vi "Realtime Monitor.vi"() -> ()   [LabVIEW 2020]
uses:
  <vilib>/Utility/sysdir.llb/System Directory Type.ctl
  <vilib>/Utility/error.llb/DialogType.ctl
  global/GlobalVariable.vi
  global/SettingVariable.vi
  <vilib>/Analysis/polynomials.llb/Scalar Polynomial Evaluation (DBL).vi
  <vilib>/Analysis/NI_AALPro.lvlib
panel:
  out "T2周期":dbl[](array[numeric]) caption="倍增周期 (s):"
  in  "拟合数":i32(knob)=5 scale=5.0..100.0
  out "实时监测趋势图":dbl[][](graph) caption="Waveform Chart - Dark"
  in  "量程衔接 2":bool
  out "量程衔接开":bool
  out "四路VO":dbl[](array[numeric]) caption="四路电压输出(V)："
  out "反应性OUT":dbl[](array[numeric])
  out "源与本底开":bool
  in  "源与本底":bool
  out "滤波开":bool
  in  "通量滤波":bool
  out "DRWM开":bool
  in  "动态刻棒":bool
  in  "量程衔接":bool
  in  "添加备注说明":string caption="添加备注说明："
  in  "Start Button":bool
  in  "停止测量":bool
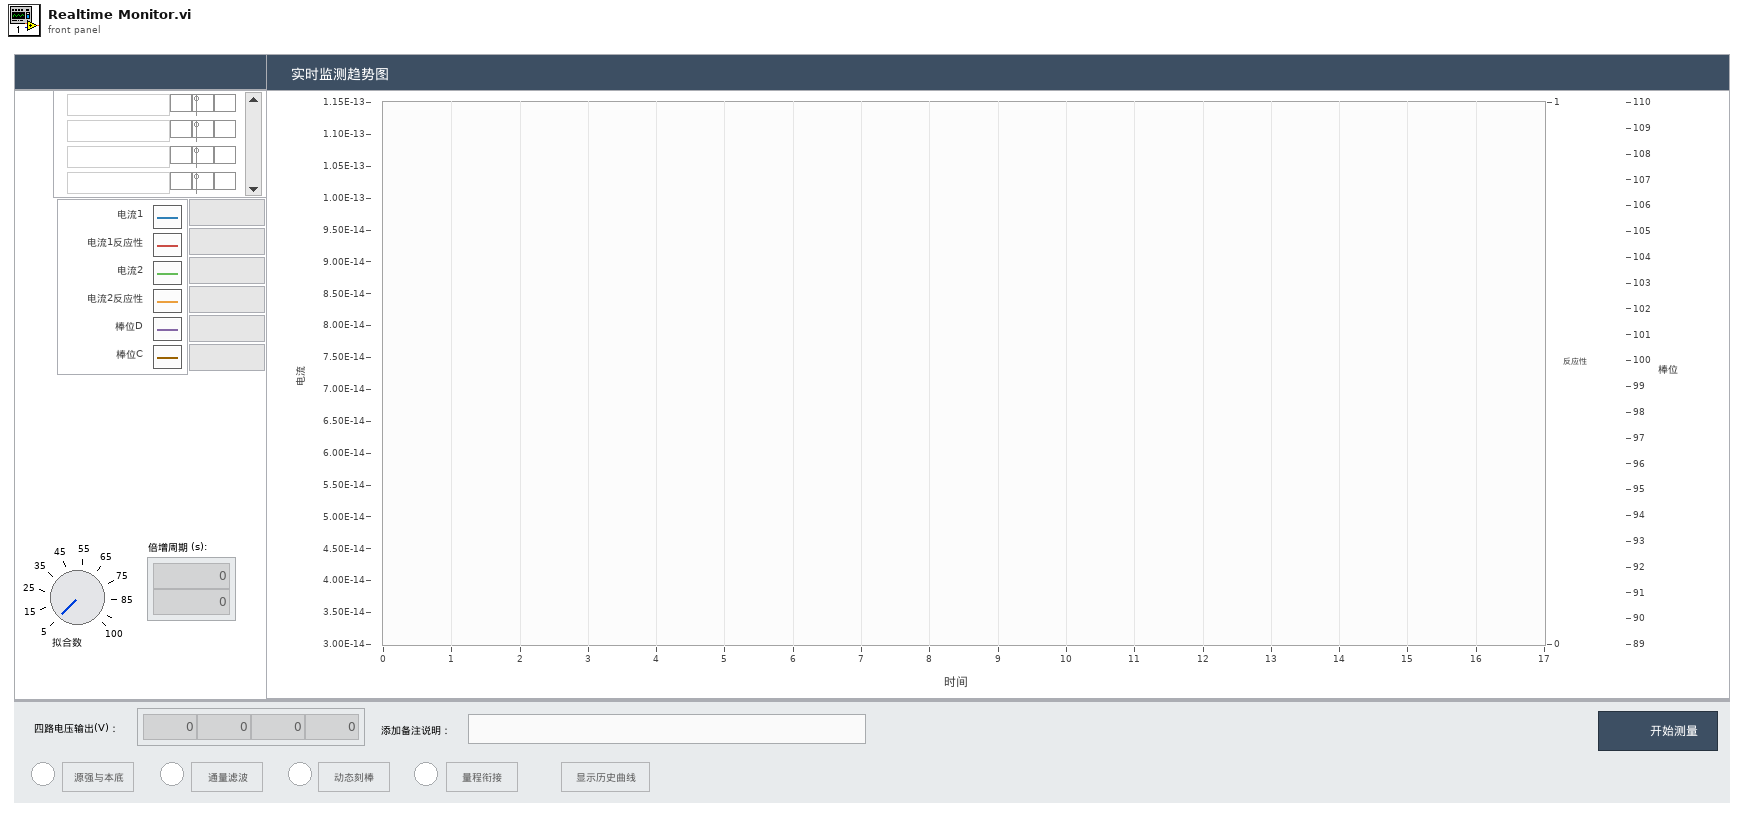
[diagram p1: front panel]
types:
  T1 = enum8{"Enabled", "Disabled", "Disabled and Grayed Out"}
  T2 = enum16{"open", "open or create", "create or replace", "create", "open (read only)"}
  T3 = cluster{"switch":bool, "name":string, "voltage upper":i32, "voltage lower":i32, "physics upper":dbl, "physics lower":dbl, "scale":u16}[]
  T4 = typedef "DialogType.ctl" = u16
  T5 = typedef "System Directory Type.ctl" = i32
  T6 = cluster{"switch":bool, "voltage upper":i32, "voltage lower":i32, "physics upper":dbl, "physics lower":dbl, "input":u16, "log":bool}[]
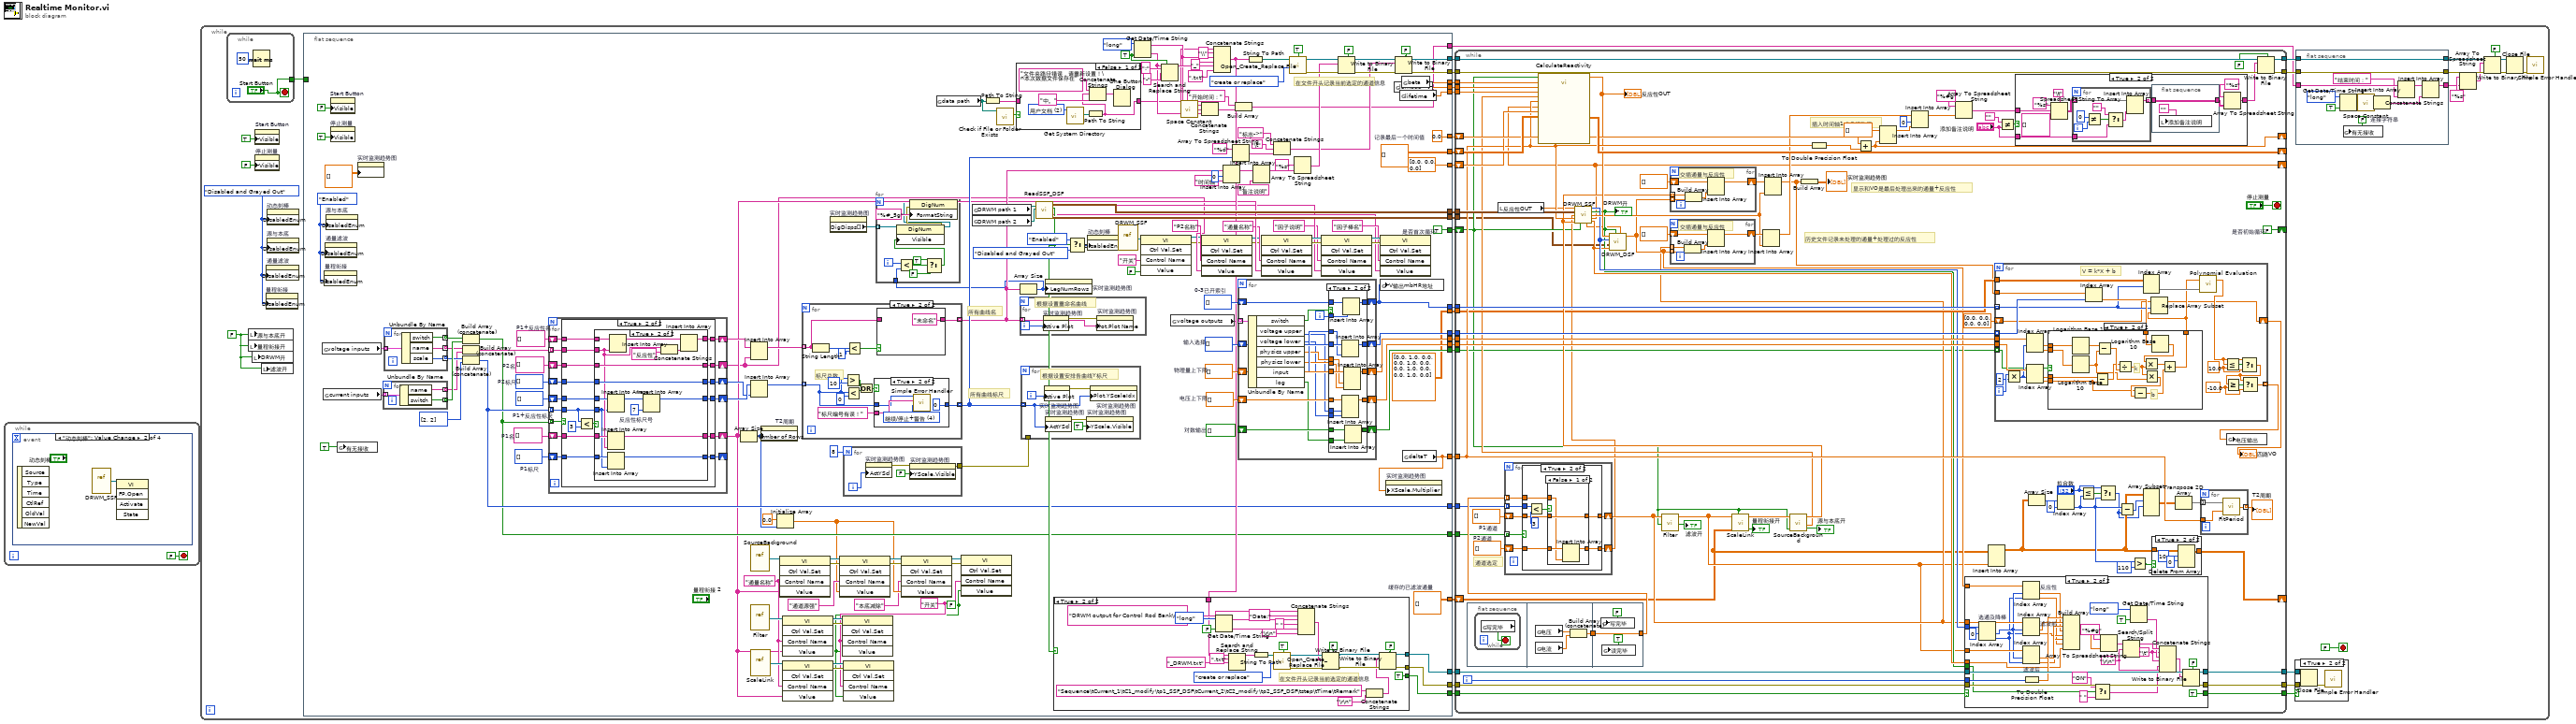
[diagram p0: block diagram]
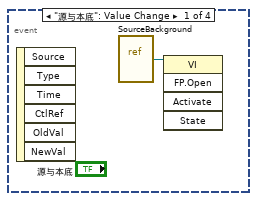
[diagram p2: hidden frame]
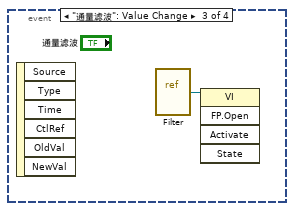
[diagram p3: hidden frame]
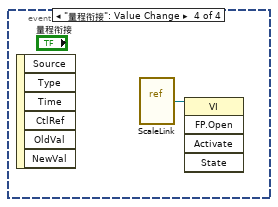
[diagram p4: hidden frame]
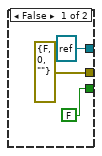
[diagram p7: hidden frame]
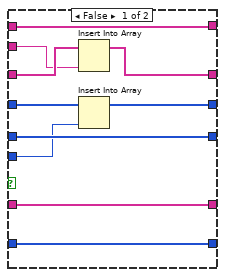
[diagram p11: hidden frame]
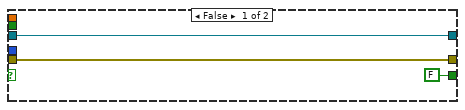
[diagram p13: hidden frame]
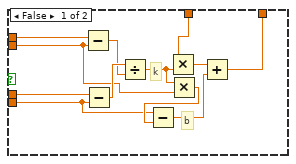
[diagram p15: hidden frame]
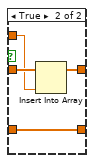
[diagram p18: hidden frame]
diagram:
  n1 = while {
    stop <- FALSE stop-if-true
    n2 = event shown="[1] \"动态刻棒\": Value Change" {
      selector: _ -> [_ _ _ _]
      dyn-events: _ -> [_ _ _ _]
      timeout: _ -> [_ _ _ _]
      event "源与本底": Value Change {
        n3 = event-data() -> ()  [unwired: 1 in, 6 out]
        n4 = vi-ref "SourceBackground.vi"() -> (w2:refnum<vi>)
        n5 = invoke class="VI" method="FP.Open"(reference=w2) -> ()  [unwired: 4 in, 5 out]
      }
      event "动态刻棒": Value Change {
        n6 = event-data() -> ()  [unwired: 1 in, 6 out]
        n7 = vi-ref "DRWM_SSF.vi"() -> (w3:refnum<vi>)
        n8 = invoke class="VI" method="FP.Open"(reference=w3) -> ()  [unwired: 4 in, 5 out]
      }
      event "通量滤波": Value Change {
        n9 = event-data() -> ()  [unwired: 1 in, 6 out]
        n10 = vi-ref "Filter.vi"() -> (w4:refnum<vi>)
        n11 = invoke class="VI" method="FP.Open"(reference=w4) -> ()  [unwired: 4 in, 5 out]
      }
      event "量程衔接": Value Change {
        n12 = event-data() -> ()  [unwired: 1 in, 6 out]
        n13 = vi-ref "ScaleLink.vi"() -> (w5:refnum<vi>)
        n14 = invoke class="VI" method="FP.Open"(reference=w5) -> ()  [unwired: 4 in, 5 out]
      }
    }
  }
  n15 = while {
    stop <- FALSE stop-if-true
    w6 = FALSE
    w7 = T1."Disabled and Grayed Out" ("Disabled")
    n16 = while {
      tunnel: ["Start Button"] -> w10
      stop <- "Start Button" stop-if-true
      n17 = Wait (ms)(milliseconds to wait=u32 50) -> ()  [unwired: 1 out]
    }
    n18 = local write "源与本底开"(w6) -> ()
    n19 = local write "量程衔接开"(w6) -> ()
    n20 = local write "DRWM开"(w6) -> ()
    n21 = property on="Start Button" class="Bool"("Visible"=TRUE) -> ()  [unwired: 2 in, 2 out]
    n22 = property on="停止测量" class="Bool"("Visible"=FALSE) -> ()  [unwired: 2 in, 2 out]
    n23 = local write "滤波开"(w6) -> ()
    n24 = property on="量程衔接" class="Bool"("DisabledEnum"=w7) -> ()  [unwired: 2 in, 2 out]
    n25 = property on="通量滤波" class="Bool"("DisabledEnum"=w7) -> ()  [unwired: 2 in, 2 out]
    n26 = property on="动态刻棒" class="Bool"("DisabledEnum"=w7) -> ()  [unwired: 2 in, 2 out]
    n27 = property on="源与本底" class="Bool"("DisabledEnum"=w7) -> ()  [unwired: 2 in, 2 out]
    n28 = flat-sequence {
      tunnel: [sgl[][] [] ("λ*Ci")] -> w50
      tunnel: [w187] -> w47
      tunnel: [w170] -> w46
      tunnel: [w169] -> w45
      tunnel: [w163] -> w44
      tunnel: [sgl[] [0.0, 0.0, 0.0] ("N(t-1)寄存")] -> w34
      tunnel: [w148] -> w33
      tunnel: [w147] -> w32
      tunnel: [w146] -> w31
      tunnel: [w145] -> w30
      tunnel: [w135] -> w29
      tunnel: [w134] -> w28
      tunnel: [w133] -> w27
      tunnel: [w132] -> w26
      tunnel: [w130] -> w23
      tunnel: [w127] -> w21
      tunnel: [w126] -> w20
      tunnel: [w125] -> w19
      tunnel: [w124] -> w18
      tunnel: [w121] -> w17
      tunnel: [w109] -> w16
      tunnel: [w108] -> w15
      tunnel: [w96] -> w14
      tunnel: [dbl[][] [[0.0, 1.0, 0.0], [0.0, 1.0, 0.0], [0.0, 1.0, 0.0], [0.0, 1.0, 0.0]]] -> w13
      tunnel: [w102] -> w12
      tunnel: w10 -> [_]
      frame #0 {
        w58 = T1."Enabled" ("Disabled")
        w59 = FALSE
        w60 = "开关" ("Control Name")
        w79 = "通量名称" ("Control Name")
        w110 = i32[] []  # P1标尺
        w111 = string[] []  # P1名
        w128 = bool[] []  # 对数输出
        w144 = i32[] []  # 0-3已开索引
        w145 = dbl[][] []  # 缓存的已滤波通量
        w149 = sgl[] []  # 电压上下限
        w150 = sgl[] []  # 物理量上下限
        w151 = u16[] []  # 输入选择
        w158 = TRUE ("需要秒？(F)")
        w163 = 0.0  # 记录最后一个时间值
        w183 = string[] []  # P2名
        w182 = i32[] []  # P2标尺
        w184 = i32[] []  # P1+反应性标尺
        w185 = string[] []  # P1+反应性名
        w187 = TRUE  # 是否首次循环
        # "所有曲线标尺"
        # "所有曲线名"
        # "在文件开头记录当前选定的通道信息"
        n29 = global read "SettingVariable.vi" "voltage inputs"() -> (w120:T3)
        n30 = global read "SettingVariable.vi" "current inputs"() -> (w119:cluster{"name":string, "switch":bool}[])
        n31 = property on="量程衔接" class="Bool"("DisabledEnum"=w58) -> ()  [unwired: 2 in, 2 out]
        n32 = property on="通量滤波" class="Bool"("DisabledEnum"=w58) -> ()  [unwired: 2 in, 2 out]
        n33 = property on="源与本底" class="Bool"("DisabledEnum"=w58) -> ()  [unwired: 2 in, 2 out]
        n34 = property on="Start Button" class="Bool"("Visible"=FALSE) -> ()  [unwired: 2 in, 2 out]
        n35 = property on="停止测量" class="Bool"("Visible"=TRUE) -> ()  [unwired: 2 in, 2 out]
        n36 = global write "GlobalVariable.vi" "有无接收"(TRUE ("写完毕")) -> ()
        n37 = property on="实时监测趋势图" class="WFChart (strict)"("History Data"=dbl[][] []) -> ()  [unwired: 2 in, 2 out]
        n38 = for {
          tunnel: w119 -> [w236] mode=indexing
          tunnel: [w235] -> w114 mode=indexing
          tunnel: [w234] -> w117 mode=indexing
          n39 = Unbundle By Name(w236) -> ("name"=w235:string, "switch"=w234:bool)
        }
        n40 = for {
          tunnel: w120 -> [w240] mode=indexing
          tunnel: [w239] -> w118 mode=indexing
          tunnel: [w238] -> w116 mode=indexing
          tunnel: [w237] -> w115 mode=indexing
          n41 = Unbundle By Name(w240) -> ("switch"=w239:bool, "name"=w238:string, "scale"=w237:u16)
        }
        n42 = Build Array (concatenate)(w118, w117) -> (w108:bool[])
        n43 = Build Array (concatenate)(w116, w114) -> (w112:string[])
        n44 = Build Array (concatenate)(w115, u16[] [2, 2] ("array")) -> (w109:u16[])
        n45 = for {
          tunnel: w112 -> [w334] mode=indexing
          shift-right: [w342] -> w181
          shift-left: w185 -> [w341]
          shift-right: [w339] -> w180
          shift-left: w184 -> [w340]
          shift-right: [w337] -> w65
          shift-left: w183 -> [w338]
          shift-right: [w335] -> w179
          shift-left: w182 -> [w336]
          tunnel: w108 -> [w333] mode=indexing
          tunnel: w109 -> [w332] mode=indexing
          shift-right: [w330] -> w74
          shift-left: w111 -> [w331]
          shift-right: [w328] -> _
          shift-left: w110 -> [w329]
          n46 = case shown="True" w333 {
            tunnel: [w348 w364] -> w342
            tunnel: w341 -> [w348 w360]
            tunnel: w334 -> [_ w359]
            tunnel: [w347 w362] -> w339
            tunnel: w340 -> [w347 w354]
            tunnel: w338 -> [w346 w358]
            tunnel: [w346 w357] -> w337
            tunnel: w336 -> [w345 w356]
            tunnel: [w345 w355] -> w335
            tunnel: w332 -> [_ w353]
            tunnel: w331 -> [w344 w352]
            tunnel: [w344 w351] -> w330
            tunnel: w329 -> [w343 w350]
            tunnel: [w343 w349] -> w328
            frame False {
            }
            frame True {
              n47 = Less?(x=w353, y=3) -> (x < y?=w361:bool)
              n48 = case shown="True" w361 {
                tunnel: w360 -> [w373 w386]
                tunnel: [w373 w391] -> w364
                tunnel: w354 -> [w374 w382]
                tunnel: [w374 w390] -> w362
                tunnel: w359 -> [w370 w379]
                tunnel: w358 -> [w372 w384]
                tunnel: [w371 w384] -> w357
                tunnel: [w367 w383] -> w355
                tunnel: w356 -> [w369 w383]
                tunnel: w353 -> [w368 w375]
                tunnel: w352 -> [w366 w380]
                tunnel: [w366 w378] -> w351
                tunnel: w350 -> [w365 w377]
                tunnel: [w365 w376] -> w349
                frame False {
                  n49 = Insert Into Array(array=w372, new element=w370) -> (w371:string[])  [unwired: 1 in]
                  n50 = Insert Into Array(array=w369, new element=w368) -> (w367:i32[])  [unwired: 1 in]
                }
                frame True {
                  w387 = 7  # 反应性标尺号
                  n51 = Insert Into Array(array=w382, new element=w375) -> (w381:i32[])  [unwired: 1 in]
                  n52 = Insert Into Array(array=w380, new element=w379) -> (w378:string[])  [unwired: 1 in]
                  n53 = Insert Into Array(array=w377, new element=w375) -> (w376:i32[])  [unwired: 1 in]
                  n54 = Insert Into Array(array=w386, new element=w379) -> (w385:string[])  [unwired: 1 in]
                  n55 = Insert Into Array(array=w381, new element=w387) -> (w390:i32[])  [unwired: 1 in]
                  n56 = Concatenate Strings(w379, "反应性" ("字符串")) -> (w388:string)
                  n57 = Insert Into Array(array=w385, new element=w388) -> (w391:string[])  [unwired: 1 in]
                }
              }
            }
          }
        }
        n58 = Array Size(array=w74) -> (size(s)=w92:i32)
        n59 = Insert Into Array(array=w181, new element=w65) -> (w177:string[])  [unwired: 1 in]
        n60 = vi-ref "SourceBackground.vi"() -> (w93:refnum<vi>)
        n61 = vi-ref "Filter.vi"() -> (w81:refnum<vi>)
        n62 = Insert Into Array(array=w180, new element=w179) -> (w178:i32[])  [unwired: 1 in]
        n63 = vi-ref "ScaleLink.vi"() -> (w80:refnum<vi>)
        n64 = property on="T2周期" class="Arr (strict)"("Number of Rows"=w92) -> ()  [unwired: 2 in, 2 out]
        n65 = Initialize Array(0.0 ("element"), w92) -> (w85:dbl[])
        n66 = invoke class="VI" method="Ctrl Val.Set"(reference=w93, "Control Name"=w79, "Value"=w74) -> (reference out=w90:refnum<vi>, error out=w89:errorcluster)  [unwired: 2 in, 3 out]
        n67 = invoke class="VI" method="Ctrl Val.Set"(reference=w81, "Control Name"=w79, "Value"=w74) -> (reference out=w64:refnum<vi>, error out=w63:errorcluster)  [unwired: 2 in, 3 out]
        n68 = invoke class="VI" method="Ctrl Val.Set"(reference=w80, "Control Name"=w79, "Value"=w74) -> (reference out=w62:refnum<vi>, error out=w61:errorcluster)  [unwired: 2 in, 3 out]
        n69 = for {
          tunnel: w178 -> [w219] mode=indexing
          tunnel: w177 -> [w216] mode=indexing
          tunnel: [w217] -> w168 mode=indexing
          tunnel: [w215] -> w143 mode=indexing
          # "标尺总数"
          n70 = String Length(string=w216) -> (length=w221:i32)
          n71 = Greater?(x=w219, y=10) -> (0:w223:bool)
          n72 = Less?(x=w219, y=0) -> (x < y?=w222:bool)
          n73 = Less?(x=w221, y=1) -> (x < y?=w214:bool)
          n74 = Or(x=w223, y=w222) -> (x .or. y?=w220:bool)
          n75 = case shown="True" w220 {
            tunnel: "标尺编号有误！" ("error source (\" \")") -> [_ w231]
            tunnel: w219 -> [w227 w230]
            tunnel: [w227 0] -> w217
            frame False {
            }
            frame True {
              w229 = T4 4 items=["无对话框", "确定信息", "继续或停止信息", "确定信息＋警告", "继续/停止+警告"] ("type of dialog (OK msg:1)")
              n76 = call <vilib>:"Simple Error Handler.vi"("error code (no error:0)"=w230, "error source (\" \")"=w231, "type of dialog (OK msg:1)"=w229) -> ()  [unwired: 2 in, 5 out]
            }
          }
          n77 = case shown="True" w214 {
            tunnel: w216 -> [w232 _]
            tunnel: [w232 "未命名"] -> w215
            frame False {
            }
            frame True {
            }
          }
        }
        n78 = property on="实时监测趋势图" class="WFChart (strict)"() -> ("DigDisps[]"=w99:refnum<vi>[])  [unwired: 2 in, 2 out]
        n79 = invoke class="VI" method="Ctrl Val.Set"(reference=w90, error in=w89, "Control Name"="通道源强", "Value"=w85) -> (reference out=w87:refnum<vi>, error out=w86:errorcluster)  [unwired: 1 in, 3 out]
        n80 = invoke class="VI" method="Ctrl Val.Set"(reference=w64, error in=w63, "Control Name"=w60, "Value"=w59) -> ()  [unwired: 1 in, 5 out]
        n81 = invoke class="VI" method="Ctrl Val.Set"(reference=w62, error in=w61, "Control Name"=w60, "Value"=w59) -> ()  [unwired: 1 in, 5 out]
        n82 = for {
          N: 8 -> [_]
          tunnel: [w201] -> w94
          i -> [w200]
          n83 = property on="实时监测趋势图" class="WFChart (strict)"("ActYScl"=w200) -> (error out=w202:errorcluster)  [unwired: 2 in, 1 out]
          n84 = property on="实时监测趋势图" class="WFChart (strict)"(error in=w202, "YScale.Visible"=FALSE ("Y Scale.Visible")) -> (error out=w201:errorcluster)  [unwired: 1 in, 1 out]
        }
        n85 = invoke class="VI" method="Ctrl Val.Set"(reference=w87, error in=w86, "Control Name"="本底减除", "Value"=w85) -> (reference out=w83:refnum<vi>, error out=w82:errorcluster)  [unwired: 1 in, 3 out]
        n86 = global read "SettingVariable.vi" "data path"() -> (w122:path)
        n87 = invoke class="VI" method="Ctrl Val.Set"(reference=w83, error in=w82, "Control Name"=w60, "Value"=w59) -> ()  [unwired: 1 in, 5 out]
        n88 = global read "SettingVariable.vi" "DRWM path 1"() -> (w104:path)
        n89 = global read "SettingVariable.vi" "DRWM path 2"() -> (w103:path)
        n90 = Path To String(path=w122) -> (string=w123:string)
        n91 = call <vilib>:"Check if File or Folder Exists.vi"("path"=w122) -> ("file or folder exists?"=w140:bool)  [unwired: 8 in, 2 out]
        n92 = case shown="False" w140 {
          tunnel: w123 -> [_ w286]
          tunnel: [w281 w286] -> w139
          frame False {
            w285 = T5 2 items=["用户目录"=0, "用户桌面"=1, "用户文档"=2, "用户应用程序数据"=3, "用户设置"=4, "用户临时目录"=5, "公共文档"=6, "公共应用程序数据"=7, "公共设置"=8, "公共缓存"=13, "系统核心库"=9, "系统安装库"=10, "应用程序文件"=11, "启动盘根目录"=12] ("system directory type")
            n93 = call <vilib>:"Get System Directory.vi"("system directory type"=w285) -> ("system directory"=w283:path)  [unwired: 10 in]
            n94 = Path To String(path=w283) -> (string=w281:string)
            n95 = Concatenate Strings("文件夹路径错误，请重新设置！\n本次数据文件保存在" ("消息"), w281, "中。" ("字符串")) -> (w284:string)
            n96 = One Button Dialog(message=w284) -> ()  [unwired: 1 in, 1 out]
          }
          frame True {
          }
        }
        n97 = for {
          tunnel: w143 -> [w247] mode=indexing
          i -> [w248]
          # "根据设置重命名曲线"
          n98 = property on="实时监测趋势图" class="WFChart (strict)"("Active Plot"=w248) -> (error out=w246:errorcluster)  [unwired: 2 in, 1 out]
          n99 = property on="实时监测趋势图" class="WFChart (strict)"(error in=w246, "Plot.Plot Name"=w247) -> ()  [unwired: 1 in, 2 out]
        }
        n100 = Array Size(array=w143) -> (size(s)=w98:i32)
        n101 = for {
          tunnel: w99 -> [w213] mode=indexing
          tunnel: w98 -> [w209]
          i -> [w211]
          n102 = Less?(x=w211, y=w209) -> (x < y?=w210:bool)
          n103 = Select(t=TRUE ("Visible"), s=w210, f=FALSE) -> (s? t:f=w207:bool)
          n104 = property class="DigNum"(reference=w213, "Visible"=w207) -> (reference out=w204:refnum<vi>, error out=w205:errorcluster)  [unwired: 1 in]
          n105 = property class="DigNum"(reference=w204, error in=w205, "FormatString"="%#_5g" ("Format String")) -> ()  [unwired: 2 out]
        }
        n106 = for {
          tunnel: w168 -> [w243] mode=indexing
          tunnel: w94 -> [_]
          i -> [w245]
          # "根据设置安排各曲线Y标尺"
          n107 = property on="实时监测趋势图" class="WFChart (strict)"("Active Plot"=w245) -> (error out=w244:errorcluster)  [unwired: 2 in, 1 out]
          n108 = property on="实时监测趋势图" class="WFChart (strict)"("ActYScl"=w243) -> (error out=w242:errorcluster)  [unwired: 2 in, 1 out]
          n109 = property on="实时监测趋势图" class="WFChart (strict)"(error in=w242, "YScale.Visible"=TRUE ("Y Scale.Visible")) -> ()  [unwired: 1 in, 2 out]
          n110 = property on="实时监测趋势图" class="WFChart (strict)"(error in=w244, "Plot.YScaleIdx"=w243) -> ()  [unwired: 1 in, 2 out]
        }
        n111 = call "ReadSSF_DSF.vi"("DRWM path 2"=w103, "DRWM path 1"=w104) -> ("DSF"=w134:cluster{"x":dbl, "y":dbl}[][], "因子棒号"=w71:string[], "SF_0K"=w129:bool, "SSF"=w135:cluster{"x":dbl, "y":dbl}[][], "文件INFO"=w70:string)  [unwired: 5 in]
        n112 = property on="实时监测趋势图" class="WFChart (strict)"("LegNumRows"=w98) -> ()  [unwired: 2 in, 2 out]
        n113 = Select(t=T1."Enabled" ("禁用"), s=w129, f=T1."Disabled and Grayed Out" ("禁用")) -> (s? t:f=w138:T1)
        n114 = property on="动态刻棒" class="Bool"("DisabledEnum"=w138) -> ()  [unwired: 2 in, 2 out]
        n115 = vi-ref "DRWM_SSF.vi"() -> (w55:refnum<vi>)
        n116 = Get Date/Time String(date format (0)=enum16{"short", "long", "abbreviated"}."long" ("日期格式(0)"), want seconds? (F)=w158) -> (date string=w156:string, time string=w155:string)  [unwired: 1 in]
        n117 = invoke class="VI" method="Ctrl Val.Set"(reference=w55, "Control Name"="开关", "Value"=FALSE) -> (reference out=w56:refnum<vi>, error out=w57:errorcluster)  [unwired: 2 in, 3 out]
        n118 = Search and Replace String(replace all?=w158, input string=w155, search string=":", replace string="-" ("replace string (\"\")")) -> (result string=w194:string)  [unwired: 4 in, 3 out]
        n119 = global read "SettingVariable.vi" "voltage outputs"() -> (w105:T6)
        n120 = call <vilib>:"Space Constant.vi"() -> ("String"=w157:string)
        n121 = Concatenate Strings ("连接字符串")(w156, w157, w155) -> (w154:string)
        n122 = invoke class="VI" method="Ctrl Val.Set"(reference=w56, error in=w57, "Control Name"="P2名称", "Value"=w65) -> (reference out=w68:refnum<vi>, error out=w67:errorcluster)  [unwired: 1 in, 3 out]
        n123 = Concatenate Strings ("连接字符串")(w139, "\\" ("字符串"), w156, "_" ("string"), w194, ".txt" ("string")) -> (w131:string)
        n124 = case shown="True" w129 {
          tunnel: [refnum<file> refnum ("refnum out") w262] -> w133
          tunnel: [errorcluster {"status"=FALSE, "code"=0, "source"=""} ("error out") w261] -> w132
          tunnel: w131 -> [_ w260]
          tunnel: [FALSE ("预置数组或字符串大小？(T)") TRUE ("预置数组或字符串大小？(T)")] -> w130
          frame False {
          }
          frame True {
            # "在文件开头记录当前选定的通道信息"
            n125 = Get Date/Time String(date format (0)=enum16{"short", "long", "abbreviated"}."long" ("日期格式(0)"), want seconds? (F)=FALSE ("需要秒？(F)")) -> (date string=w266:string, time string=w264:string)  [unwired: 1 in]
            n126 = Search and Replace String(input string=w260, search string=".txt" ("搜索字符串"), replace string="_DRWM.txt" ("字符串")) -> (result string=w257:string)  [unwired: 5 in, 3 out]
            n127 = String To Path(string=w257) -> (path=w272:path)
            n128 = call <vilib>:"Open_Create_Replace File.vi"("advisory dialog? (display:T)"=TRUE, "function (open:0)"=T2."create or replace", "file path"=w272) -> ("error out"=w279:errorcluster, "refnum"=w277:refnum<file>)  [unwired: 5 in, 2 out]
            n129 = Concatenate Strings("DRWM output for Control Rod Bank\n" ("连接的字符串"), "Date:" ("字符串"), w266, " " ("字符串"), w264, "\r\n") -> (w263:string)
            n130 = Write to Binary File(file (use dialog)=w277, data=w263, error in=w279, 5:FALSE ("预置数组或字符串大小？(T)")) -> (refnum out=w274:refnum<file>, error out=w273:errorcluster)  [unwired: 2 in, 1 out]
            n131 = Concatenate Strings("Sequence\tCurrent_1\tC1_modify\tρ1_SSF_DSF\tCurrent_2\tC2_modify\tρ2_SSF_DSF\tstep\tTime\tRemark" ("连接的字符串"), "\r\n") -> (w254:string)
            n132 = Write to Binary File(file (use dialog)=w274, data=w254, error in=w273, 5:FALSE ("预置数组或字符串大小？(T)")) -> (refnum out=w262:refnum<file>, error out=w261:errorcluster)  [unwired: 2 in, 1 out]
          }
        }
        n133 = Insert Into Array(array=w143, index=0 ("索引"), new element="时间轴" ("新元素/子数组")) -> (w162:string[])
        n134 = Array To Spreadsheet String(array=w168, 3:"%d" ("format string")) -> (spreadsheet string=w167:string)  [unwired: 1 in]
        n135 = Build Array("开始时间：" ("字符串"), w154) -> (w121:string[])
        n136 = for {
          shift-right: [w304] -> w148
          shift-left: w151 -> [w305]
          shift-right: [w300] -> w147
          shift-left: w150 -> [w301]
          shift-right: [w302] -> w146
          shift-left: w149 -> [w303]
          shift-right: [w298] -> w102
          shift-left: w144 -> [w299]
          shift-right: [w295] -> w127
          shift-left: w128 -> [w296]
          tunnel: w105 -> [w294] mode=indexing
          i -> [w297]
          n137 = Unbundle By Name(w294) -> ("switch"=w293:bool, "voltage upper"=w289:i32, "voltage lower"=w288:i32, "physics upper"=w291:dbl, "physics lower"=w290:dbl, "input"=w292:u16, "log"=w287:bool)
          n138 = case shown="True" w293 {
            tunnel: w305 -> [w310 w327]
            tunnel: [w310 w326] -> w304
            tunnel: w292 -> [_ w325]
            tunnel: w303 -> [w308 w324]
            tunnel: [w308 w323] -> w302
            tunnel: w301 -> [w309 w322]
            tunnel: [w309 w321] -> w300
            tunnel: w291 -> [_ w320]
            tunnel: w290 -> [_ w319]
            tunnel: w289 -> [_ w318]
            tunnel: w288 -> [_ w317]
            tunnel: w299 -> [w307 w316]
            tunnel: w297 -> [_ w315]
            tunnel: [w307 w314] -> w298
            tunnel: w287 -> [_ w313]
            tunnel: w296 -> [w306 w312]
            tunnel: [w306 w311] -> w295
            frame False {
            }
            frame True {
              n139 = Insert Into Array(array=w327, new element=w325) -> (w326:u16[])  [unwired: 1 in]
              n140 = Insert Into Array(array=w324, new element #1=w318, new element #2=w317) -> (w323:sgl[])  [unwired: 1 in]
              n141 = Insert Into Array(array=w316, new element=w315) -> (w314:i32[])  [unwired: 1 in]
              n142 = Insert Into Array(array=w322, new element #1=w320, new element #2=w319) -> (w321:sgl[])  [unwired: 1 in]
              n143 = Insert Into Array(array=w312, new element=w313) -> (w311:bool[])  [unwired: 1 in]
            }
          }
        }
        n144 = String To Path(string=w131) -> (path=w141:path)
        n145 = Insert Into Array(array=w162, new element="备注说明" ("新元素/子数组")) -> (w161:string[])  [unwired: 1 in]
        n146 = invoke class="VI" method="Ctrl Val.Set"(reference=w68, error in=w67, "Control Name"="通量名称", "Value"=w74) -> (reference out=w78:refnum<vi>, error out=w77:errorcluster)  [unwired: 1 in, 3 out]
        n147 = Concatenate Strings("标志->" ("字符串"), "\t", w167) -> (w164:string)
        n148 = call <vilib>:"Open_Create_Replace File.vi"("advisory dialog? (display:T)"=TRUE, "function (open:0)"=T2."create or replace", "file path"=w141) -> ("error out"=w192:errorcluster, "refnum"=w189:refnum<file>)  [unwired: 5 in, 2 out]
        n149 = Array To Spreadsheet String(array=w161, 3:"%s" ("format string")) -> (spreadsheet string=w186:string)  [unwired: 1 in]
        n150 = invoke class="VI" method="Ctrl Val.Set"(reference=w78, error in=w77, "Control Name"="因子说明", "Value"=w70) -> (reference out=w76:refnum<vi>, error out=w75:errorcluster)  [unwired: 1 in, 3 out]
        n151 = Write to Binary File(file (use dialog)=w189, data=w186, error in=w192, 5:FALSE ("预置数组或字符串大小？(T)")) -> (refnum out=w172:refnum<file>, error out=w171:errorcluster)  [unwired: 2 in, 1 out]
        n152 = invoke class="VI" method="Ctrl Val.Set"(reference=w76, error in=w75, "Control Name"="因子棒名", "Value"=w71) -> ()  [unwired: 1 in, 5 out]
        n153 = global write "GlobalVariable.vi" "V输出mbHR地址"(w102) -> ()
        n154 = global read "SettingVariable.vi" "lambda"() -> (w124:dbl[])
        n155 = Write to Binary File(file (use dialog)=w172, data=w164, error in=w171, 5:FALSE ("预置数组或字符串大小？(T)")) -> (refnum out=w170:refnum<file>, error out=w169:errorcluster)  [unwired: 2 in, 1 out]
        n156 = global read "SettingVariable.vi" "lifetime"() -> (w126:dbl)
        n157 = global read "SettingVariable.vi" "beta"() -> (w125:dbl[])
        n158 = global read "SettingVariable.vi" "deltaT"() -> (w96:dbl)
        n159 = property on="实时监测趋势图" class="WFChart (strict)"("XScale.Multiplier"=w96) -> ()  [unwired: 2 in, 2 out]
      }
    }
    n160 = while {
      shift-right: [w492] -> _
      shift-left: w50 -> [w493]
      tunnel: w19 -> [w494]
      tunnel: w18 -> [w499]
      tunnel: w20 -> [w491]
      shift-right: [w498] -> _
      shift-left: w47 -> [w409]
      tunnel: w46 -> [w490]
      tunnel: w45 -> [w497]
      tunnel: [w496] -> w49
      tunnel: w14 -> [w458]
      tunnel: [w489] -> w48
      shift-right: [w479] -> _
      shift-left: w44 -> [w482]
      shift-right: [w412] -> _
      shift-left: w34 -> [w472]
      shift-right: [w463] -> _
      shift-left: w30 -> [w432]
      tunnel: w33 -> [w467]
      tunnel: w32 -> [w466]
      tunnel: w31 -> [w465]
      tunnel: w12 -> [w464]
      tunnel: w29 -> [w460]
      tunnel: w28 -> [w408]
      tunnel: w13 -> [w450]
      tunnel: w27 -> [w448]
      tunnel: w26 -> [w447]
      tunnel: [w446] -> w25
      tunnel: [w445] -> w24
      tunnel: w23 -> [w439]
      tunnel: [w438] -> w22
      tunnel: w21 -> [w428]
      tunnel: w16 -> [w419]
      tunnel: w15 -> [w420]
      i -> [w442]
      stop <- "停止测量" stop-if-true
      w485 = dbl[] []  # P2通道
      w486 = dbl[] []  # P1通道
      w498 = FALSE  # 是否初始循环
      # "历史文件记录未处理的通量+处理过的反应性"
      # "显示和VO是最后处理出来的通量+反应性"
      # "通道选定"
      # "插入时间轴1或多行数据"
      n161 = flat-sequence {
        tunnel: [w501] -> w435
        tunnel: [w505] -> w484
        tunnel: w435 -> [w505]
        frame #0 {
          n162 = while {
            stop <- w500 stop-if-true
            n163 = global read "GlobalVariable.vi" "写完毕"() -> (w500:bool)
          }
        }
        frame #1 {
          n164 = global read "GlobalVariable.vi" "电压"() -> (w503:dbl[])
          n165 = global read "GlobalVariable.vi" "电流"() -> (w502:dbl[])
          n166 = Build Array (concatenate)(w503, w502) -> (w501:dbl[])
        }
        frame #2 {
          n167 = global write "GlobalVariable.vi" "写完毕"(FALSE ("写完毕")) -> ()
          n168 = global write "GlobalVariable.vi" "读完毕"(TRUE ("写完毕")) -> ()
        }
      }
      n169 = local read "反应性OUT"() -> (w413:dbl[])
      n170 = for {
        shift-right: [w638] -> w434
        shift-left: w486 -> [w639]
        shift-right: [w636] -> w411
        shift-left: w485 -> [w637]
        tunnel: w484 -> [w635] mode=indexing
        tunnel: w420 -> [w634] mode=indexing
        tunnel: w419 -> [w633] mode=indexing
        n171 = case shown="True" w634 {
          tunnel: w633 -> [_ w648]
          tunnel: w639 -> [w641 w646]
          tunnel: [w641 w645] -> w638
          tunnel: w637 -> [w640 w644]
          tunnel: [w640 w643] -> w636
          tunnel: w635 -> [_ w642]
          frame False {
          }
          frame True {
            n172 = Less?(x=w648, y=3) -> (x < y?=w647:bool)
            n173 = case shown="False" w647 {
              tunnel: w646 -> [w651 w656]
              tunnel: [w651 w655] -> w645
              tunnel: w644 -> [w653 w657]
              tunnel: [w652 w657] -> w643
              tunnel: w642 -> [w650 w654]
              frame False {
                n174 = Insert Into Array(array=w653, new element=w650) -> (w652:dbl[])  [unwired: 1 in]
              }
              frame True {
                n175 = Insert Into Array(array=w656, new element=w654) -> (w655:dbl[])  [unwired: 1 in]
              }
            }
          }
        }
      }
      n176 = call "Filter.vi"("首次调用"=w409, "通量in"=w434) -> ("滤波开"=→"滤波开":bool, "通量out"=w433:dbl[])  [unwired: 6 in]
      n177 = call "ScaleLink.vi"("首次调用"=w409, "曲线输入"=w432, "通量输入"=w433) -> ("开启衔接指示"=→"量程衔接开":bool, "通量输出"=w416:dbl[])  [unwired: 7 in]
      n178 = call "SourceBackground.vi"("首次调用？"=w409, "通量in"=w416) -> ("源与基线灯"=→"源与本底开":bool, "源强out"=w449:dbl[], "通量out"=w453:dbl[])  [unwired: 5 in]
      n179 = call "DRWM_SSF.vi"("反应性in"=w413, "SSF因子"=w460, "P2信号"=w411, "时间步长"=w458, "通量in"=w453, "首次调用？"=w409) -> ("上下段通量索引"=w444:u16[], "DRWM开"=w436:bool, "P2信号out"=w452:dbl[], "通量out"=w412:dbl[], "棒限"=w410:dbl[], "动态棒位"=w437:dbl)  [unwired: 4 in]
      "DRWM开" <- w436
      n180 = call "CalculateReactivity.vi"("首循环？"=w409, "λi*Ci(0)"=w493, "N(0)"=w472, "βi"=w494, "λi"=w499, "中子寿命"=w491, "源强"=w449, "采集间隔"=w458, "N(t)"=w412) -> ("λi*Ci(t)"=w492:sgl[][], "反应性OUT"=w457:dbl[])  [unwired: 5 in]
      "反应性OUT" <- w457
      n181 = call "DRWM_DSF.vi"("棒限值"=w410, "DRWM开"=w436, "动态棒位"=w437, "DSF因子"=w408, "上下段通量选择"=w444, "反应性in"=w457) -> ("反应性out"=w443:dbl[])  [unwired: 5 in]
      n182 = for {
        tunnel: w434 -> [w548] mode=indexing
        tunnel: w443 -> [w547] mode=indexing
        shift-right: [w549] -> w454
        shift-left: dbl[] [] ("平滑掉数据") -> [w550]
        # "交插通量与反应性"
        n183 = Build Array(w548, w547) -> (w546:dbl[])
        n184 = Insert Into Array(array=w550, new element=w546) -> (w549:dbl[])  [unwired: 1 in]
      }
      n185 = for {
        tunnel: w453 -> [w660] mode=indexing
        tunnel: w443 -> [w659] mode=indexing
        shift-right: [w661] -> w483
        shift-left: dbl[] [] ("平滑掉数据") -> [w662]
        # "交插通量与反应性"
        n186 = Build Array(w660, w659) -> (w658:dbl[])
        n187 = Insert Into Array(array=w662, new element=w658) -> (w661:dbl[])  [unwired: 1 in]
      }
      n188 = Insert Into Array(array=w454, new element=w452) -> (w451:dbl[])  [unwired: 1 in]
      n189 = Insert Into Array ("数组插入")(array=w483, new element=w452) -> (w430:dbl[])  [unwired: 1 in]
      n190 = Build Array(w430) -> (→"实时监测趋势图":dbl[][])
      n191 = To Double Precision Float(number=w458) -> (double precision float=w429:dbl)
      n192 = Add(x=w482, y=w429) -> (x+y=w479:dbl)
      n193 = Insert Into Array(array=dbl[] [], new element=w479) -> (w480:dbl[])  [unwired: 1 in]
      n194 = Insert Into Array(array=w451, index=0 ("索引 (行)"), new element=w480) -> (w431:dbl[])
      n195 = Array To Spreadsheet String(array=w431, 3:"%#g" ("format string")) -> (spreadsheet string=w474:string)  [unwired: 1 in]
      n196 = case shown="True" w439 {
        tunnel: w448 -> [w509 w544]
        tunnel: w447 -> [w508 w543]
        tunnel: [w509 w542] -> w446
        tunnel: [w508 w541] -> w445
        tunnel: w444 -> [_ w539]
        tunnel: w434 -> [_ w537]
        tunnel: w433 -> [_ w536]
        tunnel: w443 -> [_ w535]
        tunnel: w442 -> [_ w532]
        tunnel: [FALSE ("预置数组或字符串大小？(T)") TRUE ("预置数组或字符串大小？(T)")] -> w438
        tunnel: w437 -> [_ w510]
        tunnel: w436 -> [_ w516]
        frame False {
        }
        frame True {
          w515 = "\r\n"
          w514 = "\t"
          n197 = Index Array "选通及降棒"(array=w539, index #1=0 ("索引")) -> (element #1=w534:u16, element #2=w533:u16)  [unwired: 1 in]
          n198 = Index Array "反应性"(array=w535, index #1=w534, index #2=w533) -> (element #1=w528:dbl, element #2=w525:dbl)
          n199 = Index Array "滤波前"(array=w537, index #1=w534, index #2=w533) -> (element #1=w530:dbl, element #2=w527:dbl)
          n200 = Index Array "滤波后"(array=w536, index #1=w534, index #2=w533) -> (element #1=w529:dbl, element #2=w526:dbl)
          n201 = To Double Precision Float(number=w532) -> (double precision float=w531:dbl)
          n202 = Build Array(w531, w530, w529, w528, w527, w526, w525, w510) -> (w524:dbl[])
          n203 = Select(t="ON" ("format string"), s=w516, f=" " ("format string")) -> (s? t:f=w513:string)
          n204 = Array To Spreadsheet String(array=w524, 3:"%#g" ("format string")) -> (spreadsheet string=w522:string)  [unwired: 1 in]
          n205 = Search/Split String(string=w522, search string/char (-)=w515) -> (substring before match=w523:string)  [unwired: 1 in, 2 out]
          n206 = Get Date/Time String(date format (0)=enum16{"short", "long", "abbreviated"}."long" ("日期格式(0)"), want seconds? (F)=TRUE ("需要秒？(F)")) -> (time string=w518:string)  [unwired: 1 in, 1 out]
          n207 = Concatenate Strings(w523, w514, w518, w514, w513, w515) -> (w521:string)
          n208 = Write to Binary File(file (use dialog)=w544, data=w521, error in=w543, 5:FALSE ("预置数组或字符串大小？(T)")) -> (refnum out=w542:refnum<file>, error out=w541:errorcluster)  [unwired: 2 in, 1 out]
        }
      }
      n209 = Insert Into Array(array=w432, new element=w433) -> (w440:dbl[][])  [unwired: 2 in]
      n210 = for {
        tunnel: w467 -> [w575] mode=indexing
        tunnel: w466 -> [w581]
        tunnel: w465 -> [w580]
        tunnel: w430 -> [w576]
        tunnel: w464 -> [w559] mode=indexing
        tunnel: w450 -> [w565]
        tunnel: w428 -> [w560] mode=indexing
        tunnel: [w561] -> w427 mode=indexing
        shift-right: [w556] -> w417
        shift-left: dbl[] [0.0, 0.0, 0.0, 0.0] ("四路VO") -> [w558]
        i -> [w579]
        w567 = sgl -10.0 ("y")
        w569 = sgl 10.0 ("y")
        # "V = k*X + b"
        n211 = Multiply(x=w579, y=2) -> (x*y=w577:i32)
        n212 = Index Array(array=w581, index #1=w577) -> (element #1=w574:sgl, element #2=w571:sgl)  [unwired: 1 in]
        n213 = Index Array(array=w580, index #1=w577) -> (element #1=w572:sgl, element #2=w563:sgl)  [unwired: 1 in]
        n214 = Index Array(array=w576, index=w575) -> (element=w573:dbl)
        n215 = case shown="True" w560 {
          tunnel: w574 -> [w593 w602]
          tunnel: w573 -> [w590 w596]
          tunnel: w572 -> [w589 w598]
          tunnel: w571 -> [w587 w601]
          tunnel: w563 -> [w583 w597]
          tunnel: [w582 w594] -> w557
          frame False {
            # "b"
            # "k"
            n216 = Subtract(x=w593, y=w587) -> (x-y=w591:sgl)
            n217 = Subtract(x=w589, y=w583) -> (x-y=w592:sgl)
            n218 = Divide(x=w592, y=w591) -> (x/y=w588:sgl)
            n219 = Multiply(x=w590, y=w588) -> (x*y=w585:dbl)
            n220 = Multiply(x=w588, y=w587) -> (x*y=w586:sgl)
            n221 = Subtract(x=w583, y=w586) -> (x-y=w584:sgl)
            n222 = Add(x=w585, y=w584) -> (x+y=w582:dbl)
          }
          frame True {
            # "b"
            # "k"
            n223 = Logarithm Base 10(1:w602) -> (0:w600:sgl)
            n224 = Logarithm Base 10(1:w601) -> (0:w599:sgl)
            n225 = Subtract(x=w598, y=w597) -> (x-y=w603:sgl)
            n226 = Subtract(x=w600, y=w599) -> (x-y=w604:sgl)
            n227 = Divide(x=w603, y=w604) -> (x/y=w605:sgl)
            n228 = Multiply(x=w605, y=w599) -> (x*y=w606:sgl)
            n229 = Subtract(x=w597, y=w606) -> (x-y=w608:sgl)
            n230 = Logarithm Base 10(1:w596) -> (0:w595:dbl)
            n231 = Multiply(x=w595, y=w605) -> (x*y=w607:dbl)
            n232 = Add(x=w607, y=w608) -> (x+y=w594:dbl)
          }
        }
        n233 = Index Array(array=w565, index (row)=w559) -> (element=w564:dbl[])  [unwired: 1 in]
        n234 = Replace Array Subset(array=w558, new element=w557, index=w559) -> (w556:dbl[])
        n235 = call-poly <vilib>:"Polynomial Evaluation.vi"("P(x)"=w564, "a"=w557) -> ("P(a)"=w562:dbl)  [unwired: 1 out]
        n236 = Less Or Equal?(x=w562, y=w569) -> (x <= y?=w570:bool)
        n237 = Select(t=w562, s=w570, f=w569) -> (s? t:f=w566:dbl)
        n238 = Greater Or Equal?(x=w566, y=w567) -> (x >= y?=w568:bool)
        n239 = Select(t=w566, s=w568, f=w567) -> (s? t:f=w561:dbl)
      }
      "四路VO" <- w417
      n240 = Not Equal?(x="", y="添加备注说明") -> (x != y?=w475:bool)
      n241 = case shown="True" w475 {
        tunnel: [w612 w613] -> w473
        tunnel: "添加备注说明" -> [_ w622]
        tunnel: w474 -> [w612 w617]
        frame False {
        }
        frame True {
          n242 = Spreadsheet String To Array(delimiter (Tab)="\t", format string="%s", spreadsheet string=w617, array type (2D Dbl)=string[][] [] ("添加的数组")) -> (array=w618:string[][])
          n243 = for {
            tunnel: w618 -> [w632] mode=indexing
            tunnel: [w631] -> w616 mode=indexing
            tunnel: w622 -> [w626]
            i -> [w630]
            n244 = Not Equal?(x=0 ("y"), y=w630) -> (x != y?=w628:bool)
            n245 = Select(t="", s=w628, f=w626) -> (s? t:f=w627:string)
            n246 = Insert Into Array(array=w632, new element=w627) -> (w631:string[])  [unwired: 1 in]
          }
          n247 = flat-sequence {
            tunnel: w616 -> [w623]
            tunnel: [w623] -> w614
            frame #0 {
              n248 = local write "添加备注说明"("") -> ()
            }
          }
          n249 = Array To Spreadsheet String(array=w614, 3:"%s" ("format string")) -> (spreadsheet string=w613:string)  [unwired: 1 in]
        }
      }
      n250 = Array Size(array=w440) -> (size(s)=w471:i32[])
      n251 = Index Array(array=w471, index=0 ("索引")) -> (element=w441:i32)
      n252 = Less Or Equal?(x="拟合数", y=w441) -> (x <= y?=w469:bool)
      n253 = Select(t="拟合数", s=w469, f=w441) -> (s? t:f=w425:i32)
      n254 = Subtract(x=w441, y=w425) -> (x-y=w426:i32)
      n255 = Greater?(x=w441, y=110) -> (0:w461:bool)
      n256 = Array Subset ("数组子集")(array=w440, index (row)=w426, length (row)=w425) -> (w423:dbl[][])  [unwired: 2 in]
      n257 = case shown="True" w461 {
        tunnel: w440 -> [w551 w555]
        tunnel: [w551 w554] -> w463
        frame False {
        }
        frame True {
          n258 = Delete From Array ("删除数组元素")(array=w555, length=10 ("y"), index (row)=0 ("索引 (行)")) -> (array with subset deleted=w554:dbl[][])  [unwired: 1 in, 1 out]
        }
      }
      n259 = Transpose 2D Array(2D array=w423) -> (transposed array=w424:dbl[][])
      n260 = for {
        tunnel: w424 -> [w611] mode=indexing
        tunnel: [w609] -> w421 mode=indexing
        tunnel: w458 -> [w610]
        n261 = call "FitPeriod.vi"("delta"=w610, "curve"=w611) -> ("T2"=w609:dbl)
      }
      "T2周期" <- w421
      n262 = global write "GlobalVariable.vi" "电压输出"(w427) -> ()
      n263 = Write to Binary File(file (use dialog)=w490, data=w473, error in=w497, 5:FALSE ("预置数组或字符串大小？(T)")) -> (refnum out=w489:refnum<file>, error out=w496:errorcluster)  [unwired: 2 in, 1 out]
    }
    n264 = case shown="True" w22 {
      tunnel: w25 -> [_ w393]
      tunnel: w24 -> [_ w392]
      frame False {
      }
      frame True {
        n265 = Close File(refnum=w393, error in=w392) -> (error out=w394:errorcluster)  [unwired: 1 out]
        n266 = call <vilib>:"Simple Error Handler.vi"("error in (no error)"=w394) -> ()  [unwired: 4 in, 5 out]
      }
    }
    n267 = flat-sequence {
      tunnel: w49 -> [w401]
      tunnel: w48 -> [w402]
      tunnel: w17 -> [w400]
      tunnel: [w402] -> w38
      tunnel: [w401] -> w37
      tunnel: [w396] -> w41
      frame #0 {
        n268 = Get Date/Time String(date format (0)=enum16{"short", "long", "abbreviated"}."long" ("日期格式(0)"), want seconds? (F)=TRUE ("需要秒？(F)")) -> (date string=w405:string, time string=w404:string)  [unwired: 1 in]
        n269 = global write "GlobalVariable.vi" "有无接收"(FALSE ("写完毕")) -> ()
        n270 = call <vilib>:"Space Constant.vi"() -> ("String"=w403:string)
        n271 = Concatenate Strings "连接字符串"(w405, w403, w404) -> (w397:string)
        n272 = Insert Into Array(array=w400, new element="结束时间：" ("字符串")) -> (w398:string[])  [unwired: 1 in]
        n273 = Insert Into Array(array=w398, new element=w397) -> (w396:string[])  [unwired: 1 in]
      }
    }
    n274 = Array To Spreadsheet String(array=w41, 3:"%s" ("format string")) -> (spreadsheet string=w36:string)  [unwired: 1 in]
    n275 = Write to Binary File(file (use dialog)=w38, data=w36, error in=w37, 5:FALSE ("预置数组或字符串大小？(T)")) -> (refnum out=w40:refnum<file>, error out=w39:errorcluster)  [unwired: 2 in, 1 out]
    n276 = Close File(refnum=w40, error in=w39) -> (error out=w43:errorcluster)  [unwired: 1 out]
    n277 = call <vilib>:"Simple Error Handler.vi"("error in (no error)"=w43) -> ()  [unwired: 4 in, 5 out]
  }
